vi "RampRateCoordinated.vi"(6 "return immediately":bool, 8 "error in (no error)":T1, 10 "ramp rate":dbl, 11 "controller in":refnum<k24>) -> (0 "error out":T1, 3 "controller out":refnum<k24>)   [LabVIEW 2019]
doc: "Acceleration and Deceleration rates are set to ramp rate forcoordinated moves."
uses:
  C:/Users/patrick/Documents/GitHub/Aerotech-Delay-Line/lvsrc/Aerotech-Ensemble-LabVIEW/2010-5.6/Bin/Aerotech.Ensemble.dll
  Bin/Aerotech.Ensemble.dll
  C:/Users/patrick/Documents/GitHub/Aerotech-Delay-Line/lvsrc/Aerotech-Ensemble-LabVIEW/2010-5.6/Bin/Aerotech.Ensemble.LabVIEW.dll
  Bin/Aerotech.Ensemble.LabVIEW.dll
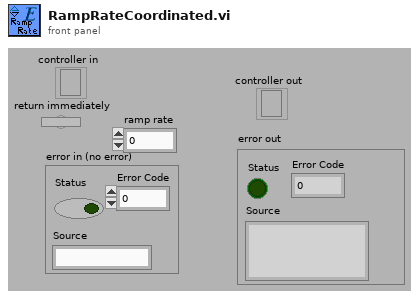
[diagram p1: front panel]
types:
  T1 = cluster{"Status":bool, "Error Code":i32, "Source":string}
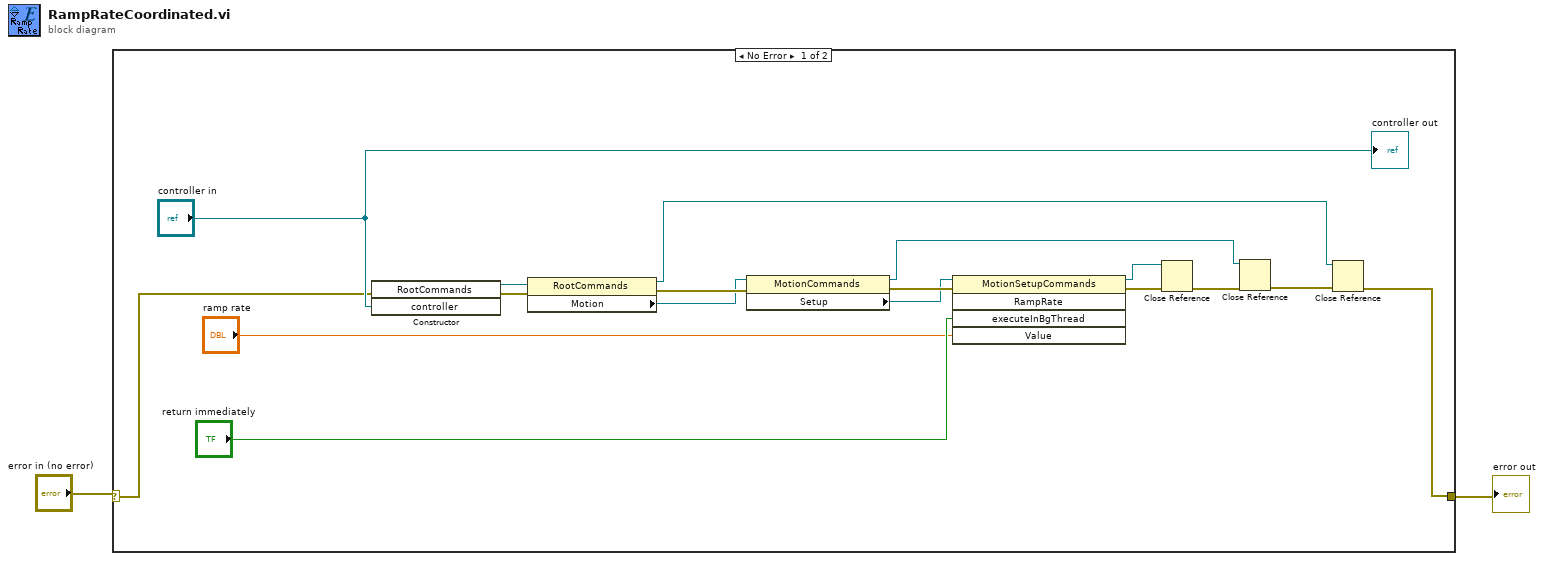
[diagram p0: block diagram]
diagram:
  n1 = case shown="No Error" "error in (no error)" {
    selector: "error in (no error)" -> [w3 w20]
    tunnel: [w7 w20] -> w1
    frame No Error {
      n2 = constructor class="RootCommands"(error in=w3, "controller"="controller in") -> (reference out=w19:refnum<k24>, error out=w18:errorcluster)  [unwired: 2 in, 2 out]
      n3 = property class="RootCommands"(reference=w19, error in=w18) -> (reference out=w8:refnum<k24>, error out=w17:errorcluster, "Motion"=w16:refnum<k24>)
      n4 = property class="MotionCommands"(reference=w16, error in=w17) -> (reference out=w10:refnum<k24>, error out=w15:errorcluster, "Setup"=w14:refnum<k24>)
      n5 = invoke class="MotionSetupCommands" method="RampRate"(reference=w14, error in=w15, "executeInBgThread"="return immediately", "Value"="ramp rate") -> (reference out=w12:refnum<k24>, error out=w13:errorcluster)  [unwired: 1 in, 3 out]
      n6 = Close Reference(reference=w12, error in (no error)=w13) -> (error out=w11:errorcluster)
      n7 = Close Reference(reference=w10, error in (no error)=w11) -> (error out=w9:errorcluster)
      n8 = Close Reference(reference=w8, error in (no error)=w9) -> (error out=w7:errorcluster)
      "controller out" <- "controller in"
    }
    frame Error {
    }
  }
  "error out" <- w1
